vi "Read Synapses.vi"(11 "Synapses in":refnum<class "Synapses.lvclass">) -> (0 "Name synapses File":string, 1 "Synapses":T1[](array[typedef]), 2 "Name grid Parent":string, 3 "Synapses out":refnum<class "Synapses.lvclass">)   [LabVIEW 2013, in "Synapses.lvclass"]
uses:
  Synapses.lvclass
  Controls/Synapses.ctl
  Controls/Type of Synapses.ctl
  Synapses.lvclass/Synapses.ctl
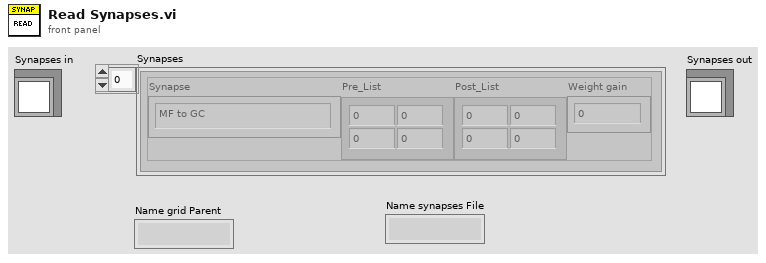
[diagram p1: front panel]
types:
  T1 = typedef "Synapses.ctl" = cluster{"Synapse":T2, "Pre_List":i32[][], "Post_List":i32[][], "Weight gain":dbl}
  T2 = typedef "Type of Synapses.ctl" = enum16{"MF to GC", "GO to GC", "GC to GO", "MF to GO", "GC to PC", "GC to BA", "PC to BA", "BA to PC", "BA to GO"}
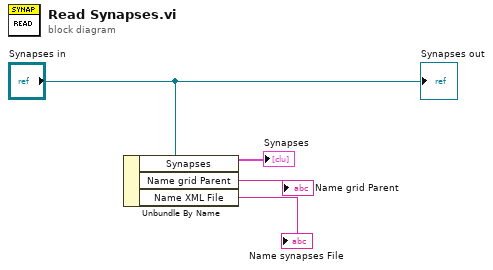
[diagram p0: block diagram]
diagram:
  n1 = Unbundle By Name("Synapses in") -> ("Synapses"=→"Synapses":T1[], "Name grid Parent"=→"Name grid Parent":string, "Name XML File"=→"Name synapses File":string)
  "Synapses out" <- "Synapses in"
